vi "Terminal_Drive_Syetem_Display.vi"   [LabVIEW 2014]
types:
  T1 = cluster{"变送器配电模块电压":u16, "变频器电流":u16, "变频器电压":u16, "变频器频率":u16, "动力子系统状态字":cluster{"电机温度过高报警":bool, "变频器电气参数异常报警":bool, "电机过载报警":bool, "电机转速误差过大报警":bool}}
  T2 = cluster{"电机温度过高报警":bool, "变频器电气参数异常报警":bool, "电机过载报警":bool, "电机转速误差过大报警":bool}
  T3 = cluster{cluster{sgl, sgl, "变送器配电模块电压":u16}, cluster{sgl, sgl, "变频器电流":u16}, cluster{sgl, sgl, "变频器电压":u16}, cluster{sgl, sgl, "变频器频率":u16}, "动力子系统状态字":cluster{"电机温度过高报警":bool, "变频器电气参数异常报警":bool, "电机过载报警":bool, "电机转速误差过大报警":bool}}
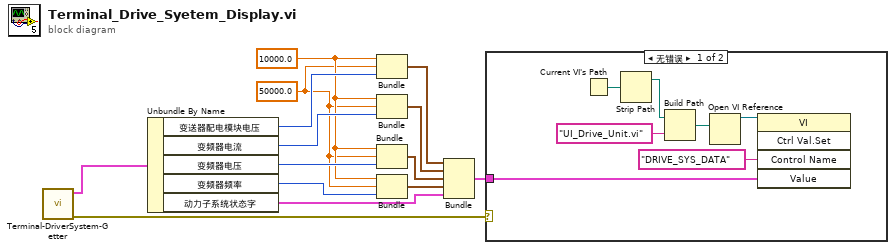
[diagram p0: block diagram]
diagram:
  w8 = sgl 50000.0
  w9 = sgl 10000.0
  n1 = call "Terminal-DriverSystem-Getter.vi"() -> ("error out"=w1:errorcluster, "设备信息"=w14:T1)  [unwired: 10 in]
  n2 = Unbundle By Name(w14) -> ("变送器配电模块电压"=w13:u16, "变频器电流"=w12:u16, "变频器电压"=w11:u16, "变频器频率"=w10:u16, "动力子系统状态字"=w3:T2)
  n3 = Bundle(w9, w8, "变送器配电模块电压"=w13) -> (w7:cluster{sgl, sgl, "变送器配电模块电压":u16})  [unwired: 1 in]
  n4 = Bundle(w9, w8, "变频器电流"=w12) -> (w6:cluster{sgl, sgl, "变频器电流":u16})  [unwired: 1 in]
  n5 = Bundle(w9, w8, "变频器电压"=w11) -> (w5:cluster{sgl, sgl, "变频器电压":u16})  [unwired: 1 in]
  n6 = Bundle(w9, w8, "变频器频率"=w10) -> (w4:cluster{sgl, sgl, "变频器频率":u16})  [unwired: 1 in]
  n7 = Bundle(w7, w6, w5, w4, "动力子系统状态字"=w3) -> (w2:T3)  [unwired: 1 in]
  n8 = case shown="无错误" w1 {
    tunnel: w2 -> [w15 _]
    frame No Error {
      n9 = Current VI's Path() -> (path=w19:path)
      n10 = Strip Path(path=w19) -> (stripped path=w20:path)  [unwired: 1 out]
      n11 = Build Path(base path=w20, name or relative path="UI_Drive_Unit.vi") -> (appended path=w17:path)
      n12 = Open VI Reference(vi path=w17) -> (vi reference=w16:refnum<vi>)  [unwired: 5 in, 1 out]
      n13 = invoke class="VI" method="Ctrl Val.Set"(reference=w16, "Control Name"="DRIVE_SYS_DATA", "Value"=w15) -> ()  [unwired: 2 in, 5 out]
    }
    frame Error {
    }
  }
